vi "Update-image-offsets.vi"(8 "error in (no error)":errorcluster, 11 "Data ref. in":refnum<data-value>) -> (0 "error out":errorcluster, 1 "Y-offsets":i32[](array[numeric]), 2 "X-offsets":i32[](array[numeric]), 3 "Data ref.":refnum<data-value>, 5 "Succes?":bool)   [LabVIEW 2013, in "CameraVision.lvlib" / "CV-Main.lvclass"]
uses:
  CV-Main.lvclass
  UI/Popup-messages.ctl
  CV-Main.lvclass/CV-Main.ctl
  Configuration/CV-Configuration.lvclass/CV-Configuration.ctl
  Read Config params.vi
  Configuration/Read Camport array.vi
  Configuration/Read ROI width.vi
  Configuration/Read ROI height.vi
  Configuration/Read Center X cam. 1.vi
  Configuration/Read Center Y cam. 1.vi
  Configuration/Read Center X cam. 2.vi
  Configuration/Read Center Y cam. 2.vi
  Configuration/Write X-offsets.vi
  Configuration/Write Y-offsets.vi
  Configuration/CV-Configuration.lvclass
  UI/CV-UI.lvclass
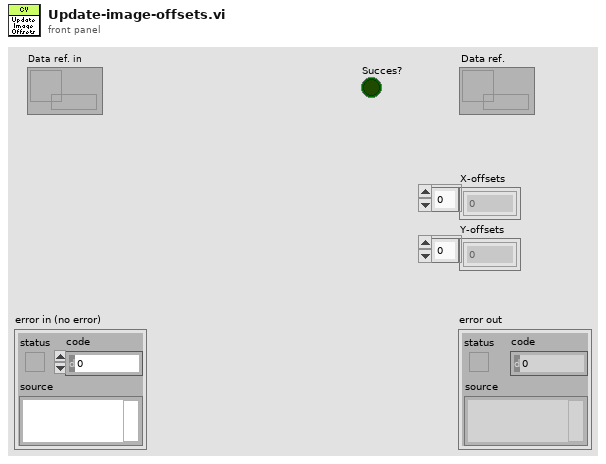
[diagram p1: front panel]
types:
  T1 = typedef "CameraVision.lvlib/CV-UI.lvclass/Popup-messages.ctl" = enum16{"Error-Black image", "Error-Camera config file", "Error-Camera connect", "Error-Grabber init", "Error-Camera setting", "Error-Image offset", "Error-Image import", "Error-Settings file not exist", "Error-Timing source", "Conflict-Filters", "Conflict-Map", "Conflict-Framerate", "Conflict-Charact", "Conflict-Temperature field", "Conflict-Temperature value", "Conflict-Storage-Binary image", "Conflict-Storage-Corrected image", "Conflict-Storage-Map", "Conflict-Storage-Charact", "Conflict-Storage-Temperature field", "Conflict-Storage-Temperature value", "Warning-File exist", "Warning-Parameter reset", "Warning-User cancel", "Info-Images imported"}
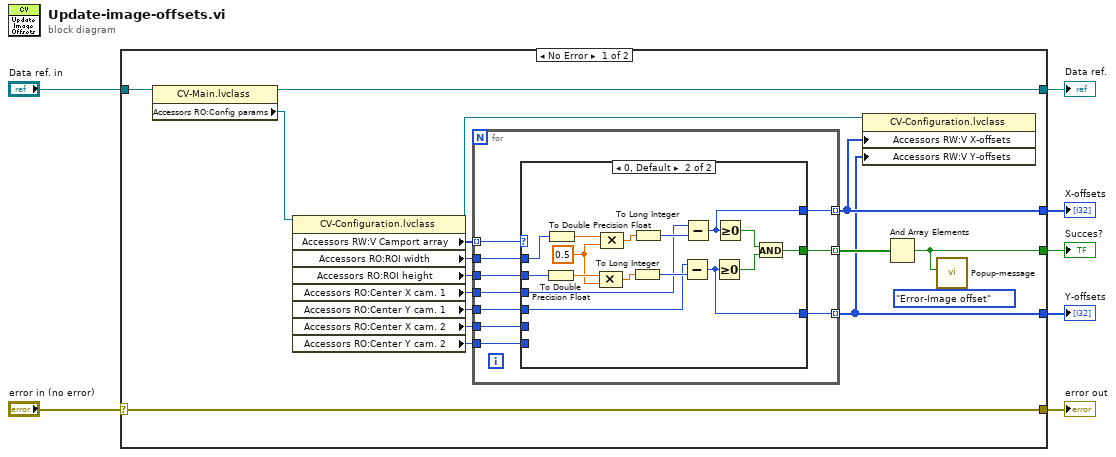
[diagram p0: block diagram]
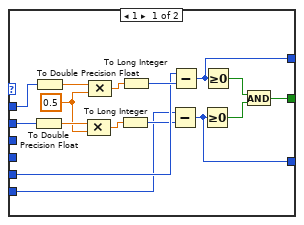
[diagram p2: hidden frame]
diagram:
  n1 = case shown="No Error" "error in (no error)" {
    selector: "error in (no error)" -> [w14 w68]
    tunnel: [w14 w68] -> w6
    tunnel: "Data ref. in" -> [w24 w67]
    tunnel: [w15 w67] -> w4
    tunnel: [w11 _] -> w3
    tunnel: [w10 _] -> w2
    tunnel: [w9 _] -> w1
    frame No Error {
      n2 = property class="CV-Main.lvclass"(reference=w24) -> (reference out=w15:refnum<data-value>, "Accessors RO:Config params"=w23:refnum<data-value>)  [unwired: 1 in, 1 out]
      n3 = property class="CV-Configuration.lvclass"(reference=w23) -> (reference out=w12:refnum<data-value>, "Accessors RW:V Camport array"=w22:u32[], "Accessors RO:ROI width"=w21:u32, "Accessors RO:ROI height"=w20:u32, "Accessors RO:Center X cam. 1"=w19:i32, "Accessors RO:Center Y cam. 1"=w18:i32, "Accessors RO:Center X cam. 2"=w17:i32, "Accessors RO:Center Y cam. 2"=w16:i32)  [unwired: 1 in, 1 out]
      n4 = for {
        tunnel: w22 -> [w34] mode=indexing
        tunnel: w21 -> [w33]
        tunnel: w20 -> [w32]
        tunnel: w19 -> [w31]
        tunnel: w18 -> [w30]
        tunnel: w17 -> [w29]
        tunnel: w16 -> [w28]
        tunnel: [w27] -> w10 mode=indexing
        tunnel: [w26] -> w9 mode=indexing
        tunnel: [w25] -> w13 mode=indexing
        n5 = case shown="0, Default" w34 {
          tunnel: w33 -> [w47 w63]
          tunnel: w32 -> [w40 w58]
          tunnel: w31 -> [_ w55]
          tunnel: w30 -> [_ w54]
          tunnel: w29 -> [w46 _]
          tunnel: w28 -> [w41 _]
          tunnel: [w37 w53] -> w25
          tunnel: [w36 w52] -> w27
          tunnel: [w35 w51] -> w26
          frame 1 {
            w42 = 0.5
            n6 = To Double Precision Float(number=w40) -> (double precision float=w44:dbl)
            n7 = To Double Precision Float(number=w47) -> (double precision float=w49:dbl)
            n8 = Compound Arithmetic op=MULTIPLY(w44, w42) -> (w43:dbl)
            n9 = Compound Arithmetic op=MULTIPLY(w49, w42) -> (w50:dbl)
            n10 = To Long Integer(number=w43) -> (32bit integer=w45:i32)
            n11 = To Long Integer(number=w50) -> (32bit integer=w48:i32)
            n12 = Subtract(x=w41, y=w45) -> (x-y=w35:i32)
            n13 = Subtract(x=w46, y=w48) -> (x-y=w36:i32)
            n14 = Greater Or Equal To 0?(x=w35) -> (x >= 0?=w38:bool)
            n15 = Greater Or Equal To 0?(x=w36) -> (x >= 0?=w39:bool)
            n16 = And(x=w39, y=w38) -> (x .and. y?=w37:bool)
          }
          frame 0, Default {
            w59 = 0.5
            n17 = To Double Precision Float(number=w58) -> (double precision float=w61:dbl)
            n18 = To Double Precision Float(number=w63) -> (double precision float=w65:dbl)
            n19 = Compound Arithmetic op=MULTIPLY(w61, w59) -> (w60:dbl)
            n20 = Compound Arithmetic op=MULTIPLY(w65, w59) -> (w66:dbl)
            n21 = To Long Integer(number=w60) -> (32bit integer=w62:i32)
            n22 = To Long Integer(number=w66) -> (32bit integer=w64:i32)
            n23 = Subtract(x=w54, y=w62) -> (x-y=w51:i32)
            n24 = Subtract(x=w55, y=w64) -> (x-y=w52:i32)
            n25 = Greater Or Equal To 0?(x=w51) -> (x >= 0?=w56:bool)
            n26 = Greater Or Equal To 0?(x=w52) -> (x >= 0?=w57:bool)
            n27 = And(x=w57, y=w56) -> (x .and. y?=w53:bool)
          }
        }
      }
      n28 = property class="CV-Configuration.lvclass"(reference=w12, "Accessors RW:V X-offsets"=w10, "Accessors RW:V Y-offsets"=w9) -> ()  [unwired: 1 in, 2 out]
      n29 = And Array Elements(Boolean array=w13) -> (logical AND=w11:bool)
      n30 = call "Popup-message.vi"("Message"=Popup-messages."Error-Image offset", "Ignore?"=w11) -> ()  [unwired: 9 in, 1 out]
    }
    frame Error {
    }
  }
  "error out" <- w6
  "Data ref." <- w4
  "Succes?" <- w3
  "X-offsets" <- w2
  "Y-offsets" <- w1
